vi "CreateEmptyImageGreyscale.vi"(7 "Value (Default: 0)":u8, 8 "error in (no error)":errorcluster, 11 "Preallocated Image Size (Default 0,0)":T1) -> (0 "error out":errorcluster, 3 "New Greyscale Image":refnum<data-value>)   [LabVIEW 2020, in "g_ar_toolkit.image.lvlib"]
uses:
  g_ar_toolkit.image.lvlib
  g_ar_toolkit.common/Image Size (Integer).ctl
  6598b9e0-8a08-46f5-91fd-ca1b87217137.vi
  <vilib>/Utility/error.llb/Error Cluster From Error Code.vi
  g_ar_toolkit.common/g_ar_toolkit.common.lvlib
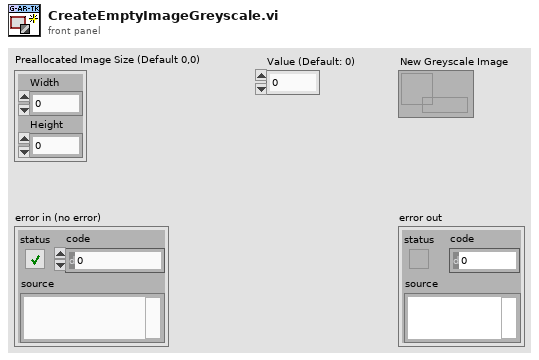
[diagram p1: front panel]
types:
  T1 = typedef "g_ar_toolkit.common.lvlib/Image Size (Integer).ctl" = cluster{"Width":u16, "Height":u16}
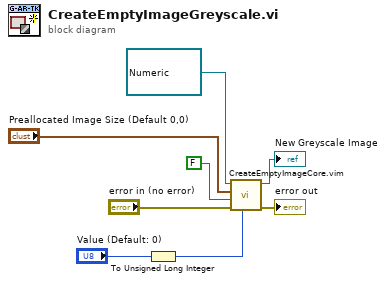
[diagram p0: block diagram]
diagram:
  n1 = To Unsigned Long Integer(number="Value (Default: 0)") -> (unsigned 32bit integer=w1:u32)
  n2 = call "CreateEmptyImageCore.vim"("Initial Value"=w1, "error in (no error)"="error in (no error)", "Is ARGB"=FALSE, "Preallocated Image Size"="Preallocated Image Size (Default 0,0)", "Ref Type"=refnum<data-value> refnum ("EDVR")) -> ("error out"=→"error out":errorcluster, "New Reference"=→"New Greyscale Image":refnum<data-value>)  [unwired: 5 in]
